vi "Executor.vi"(0 "DevControl 输入":refnum<class "DevControl.lvclass"> caption="DNL_LabVIEW Object in", 5 "Addr":u8, 7 "DevCmd":T1 items=["WriteAddr"=81, "Enable"=80, "Red"=66, "Green"=65, "TurnOn"=49, "Shutdown"=48, "GetESD"=34], 9 "Data":u8, 11 "error in (no error)":errorcluster caption="错误输入（无错误）", 12 "ChkDat?":bool=TRUE) -> (4 "DevControl 输出":refnum<class "DevControl.lvclass"> caption="DNL_LabVIEW Object out", 8 "Data":u8, 15 "error out":errorcluster caption="错误输出")   [LabVIEW 2012, in "DevControl.lvclass"]
uses:
  DevControl.lvclass
  SupportVi/DevCmd.ctl
  DevControl.lvclass/DevControl.ctl
  Libs/Serial/Serial.lvclass
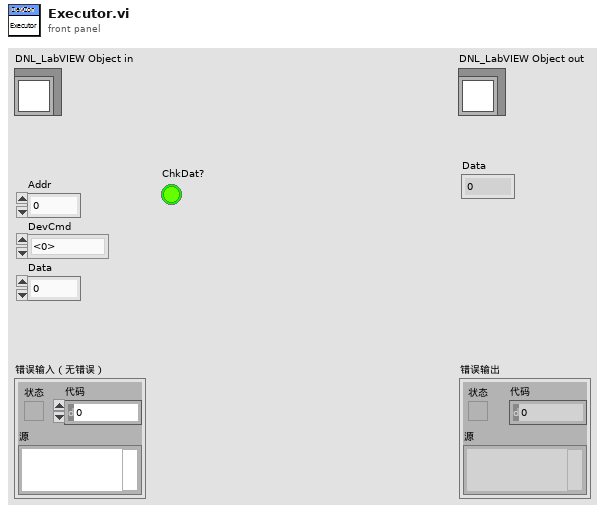
[diagram p1: front panel]
types:
  T1 = typedef "DevControl.lvclass/DevCmd.ctl" = u8
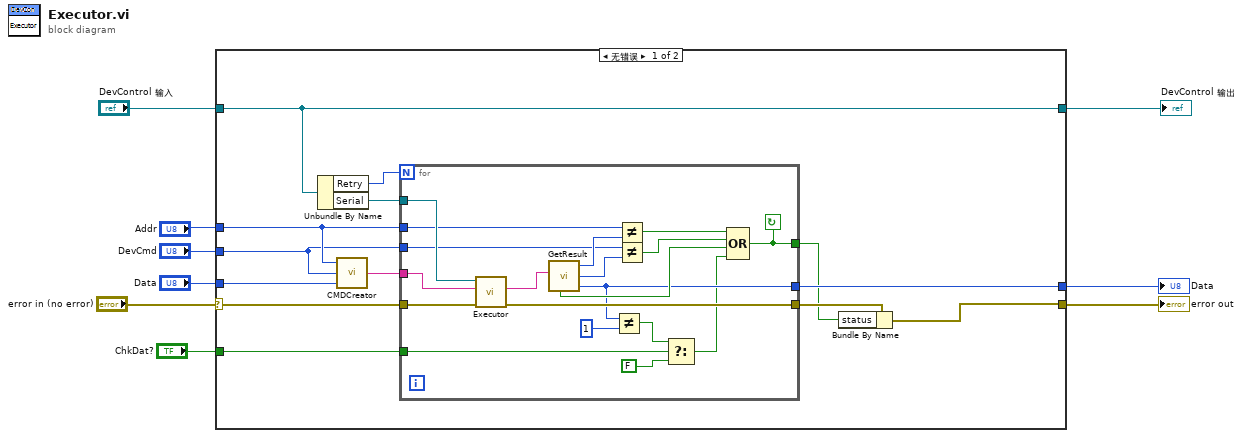
[diagram p0: block diagram]
diagram:
  n1 = case shown="无错误" "error in (no error)" {
    selector: "error in (no error)" -> [w22 w43]
    tunnel: [w12 w43] -> w8
    tunnel: [w21 w42] -> w6
    tunnel: "DevControl 输入" -> [w21 w42]
    tunnel: "Addr" -> [w18 _]
    tunnel: "DevCmd" -> [w17 _]
    tunnel: [w15 _] -> w3
    tunnel: "Data" -> [w16 _]
    tunnel: "ChkDat?" -> [w14 _]
    frame No Error {
      n2 = Unbundle By Name(w21) -> ("Retry"=w13:i32, "Serial"=w20:refnum<class "Serial.lvclass">)
      n3 = call "CMDCreator.vi"("Data"=w16, "DevCmd"=w17, "Addr"=w18) -> ("Buff"=w19:string)  [unwired: 2 in]
      n4 = for {
        N: w13 -> [_]
        tunnel: w22 -> [w41]
        tunnel: w20 -> [w40]
        tunnel: w19 -> [w39]
        tunnel: [w37] -> w11
        tunnel: w18 -> [w36]
        tunnel: w17 -> [w34]
        tunnel: [w23] -> w10
        tunnel: [w29] -> w15
        tunnel: w14 -> [w27]
        stop <- w23 continue-if-true
        n5 = call-dynamic "Executor.vi"("error in (no error)"=w41, "WriteBuff"=w39, "Serial 输入"=w40) -> ("error out"=w37:errorcluster, "ReadBuf"=w38:string)  [unwired: 5 in, 2 out]
        n6 = call "GetResult.vi"("ReadBuff"=w38) -> ("Error?"=w30:bool, "Addr"=w35:u8, "Cmd"=w33:u8, "Data"=w29:u8)  [unwired: 4 in]
        n7 = Not Equal?(x=w29, y=u8 1) -> (x != y?=w26:bool)
        n8 = Not Equal?(x=w36, y=w35) -> (x != y?=w32:bool)
        n9 = Not Equal?(x=w34, y=w33) -> (x != y?=w31:bool)
        n10 = Select(t=w26, s=w27, f=FALSE) -> (s? t:f=w24:bool)
        n11 = Compound Arithmetic op=OR(w32, w31, w30, w24) -> (w23:bool)
      }
      n12 = Bundle By Name(cluster=w11, "status"=w10) -> (w12:errorcluster)
    }
    frame Error {
    }
  }
  "error out" <- w8
  "DevControl 输出" <- w6
  "Data" <- w3
